vi "Material-ConvertTo-Dbl.vi"(0 "DBL String":string) -> (6 "DBL liner out":dbl)   [LabVIEW 2013, in "Material-RunTest.lvclass"]
uses:
  Material-RunTest.lvclass
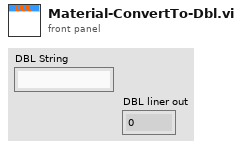
[diagram p1: front panel]
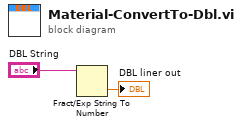
[diagram p0: block diagram]
diagram:
  n1 = Fract/Exp String To Number(string="DBL String") -> (number=→"DBL liner out":dbl)  [unwired: 3 in, 1 out]
